vi "Client_02.vi"() -> ()   [LabVIEW 2010]
doc: "Demonstrates how to display an interactive send and receive message dialog for communication between TCP connections. It establishes a connection on the machine listed and the port specified. It then waits for you to input data into the Input Line string control and hit enter. Once you hit enter, the string you typed is sent to the port and passed to the TCP Communicator - Passive.vi where it is displayed on a string indicator.\n\nThe key difference between the Active and Passive VIs is that the Active VI establishes a connection, while the Passive VI waits for a connection to be established.\n\n<B>Note:</B> Requires the TCP Communicator - Passive.vi."
panel:
  out "warning out":errorcluster
  in  "Port":u16=12673
  in  "Machine":string="ssh.alwaysdata.com"
  out "Their Response:":string
  in  "stop":bool
  out "You Typed:":string
  in  "Input Line":string
  # "Instructions:\n1. Open the TCP\n    Communicator - Passive.vi\n    and run it first.\n2. Run TCP Communicator - \n    Active.vi second.\n3.Type into the Input Line\n    String Control and then\n    hit Enter.\n4. Type into the Input Line\n    of the other VI and then\n    hit Enter.\n5. Press Stop to end session."
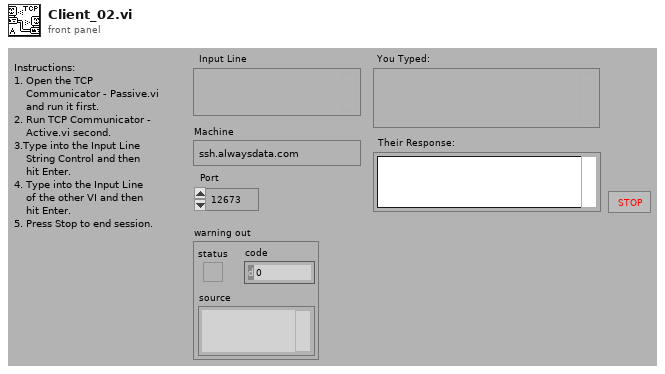
[diagram p1: front panel]
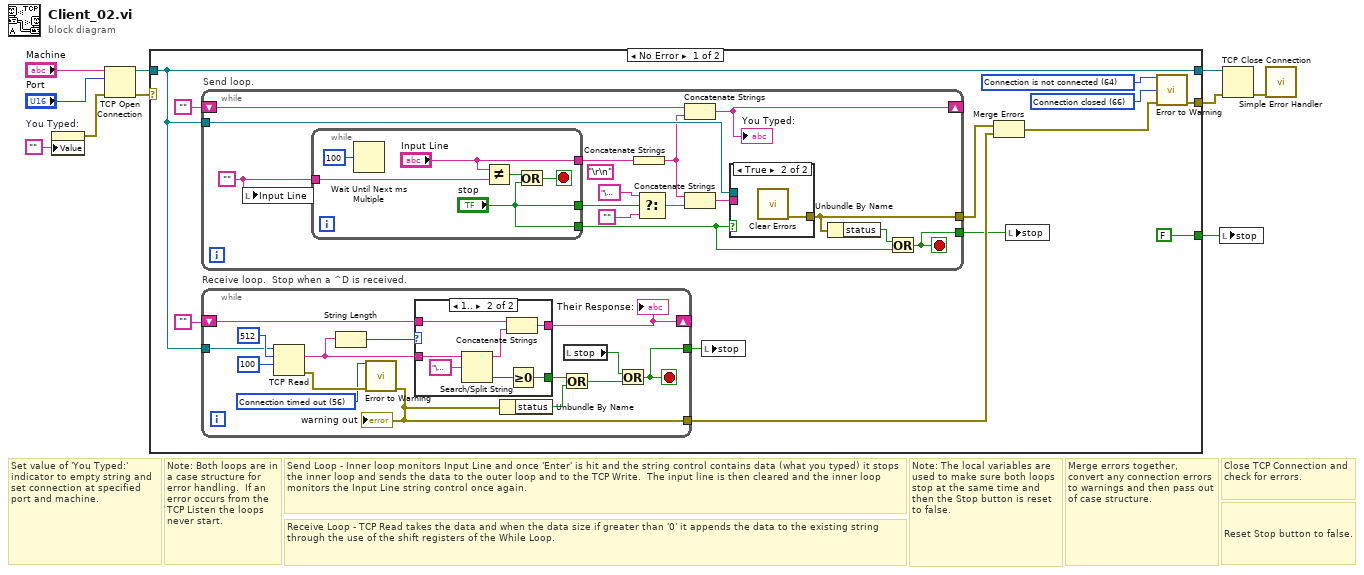
[diagram p0: block diagram]
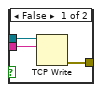
[diagram p2: hidden frame]
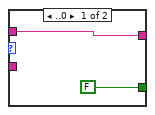
[diagram p3: hidden frame]
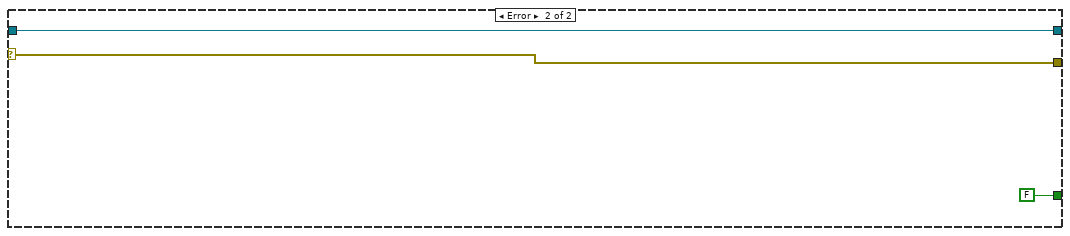
[diagram p4: hidden frame]
diagram:
  # "Set value of 'You Typed:' indicator to empty string and set connection at specified port and machine."
  # "Send Loop - Inner loop monitors Input Line and once 'Enter' is hit and the string control contains data (what you typed) it stops the inner loop and sends the data to the outer loop and to the TCP Write.  The input line is then cleared and the inner loop monitors the Input Line string control once again."
  # "Receive Loop - TCP Read takes the data and when the data size if greater than '0' it appends the data to the existing string through the use of the shift registers of the While Loop."
  # "Note: The local variables are used to make sure both loops stop at the same time and then the Stop button is reset to false."
  # "Merge errors together, convert any connection errors to warnings and then pass out of case structure."
  # "Note: Both loops are in a case structure for error handling.  If an error occurs from the TCP Listen the loops never start."
  # "Close TCP Connection and check for errors."
  # "Reset Stop button to false."
  n1 = property on="You Typed:" class="Str"("Value"="") -> (error out=w5:errorcluster)  [unwired: 2 in, 1 out]
  n2 = TCP Open Connection(address="Machine", remote port or service name="Port", error in (no error)=w5) -> (connection ID=w7:refnum<k5>, error out=w8:errorcluster)  [unwired: 2 in]
  n3 = case shown="No Error" w8 {
    selector: w8 -> [_ w73]
    tunnel: [w14 w73] -> w3
    tunnel: w7 -> [w20 w74]
    tunnel: [w20 w74] -> w4
    tunnel: [FALSE FALSE] -> w1
    frame No Error {
      w15 = 66 items=["No Error", "Argument Error", "Memory Full", "Out of Zone", "End of File", "File Already Open", "Generic File IO Error", "File Not Found", "File Permission Error", "Disk Full", "Duplicate Path", "Too Many Files Open", "Not Enabled", "Resource File Not Found", "Cannot Add Resource", "Resource Not Found", "Image Not Found", "Image Memory Error", "Pen Does Not Exist", "Config Bad Type", "Config Token Not Found", "Config Parse Error", "Config Memory Error", "Bad External Code Format", "Bad External Code Offset", "External Code Not Present", "Null Window", "Destroy Window Mixup", "Null Menu", "Print Aborted", "Bad Print Record", "Print Driver Error", "Windows Error During Print", "Memory Error During Print", "Print Dialog Error", "Generic Print Error", "Invalid Device Refnum", "Device Not Found", "Device Parameter Error", "Device Unit Error", "Can't Open Device", "Device Call Aborted", "Generic Error", "Cancelled By User", "Object ID Too Low", "Object ID Too High", "Object Not In Heap", "Unknown Heap", "Bad DefProc ID", "DefProc Not In Table", "Message Out Of Range", "Null Method", "Unknown Message", "Manager Call Not Supported", "Bad address", "Connection In progress", "Connection timed out", "Connection is already in progress", "Network attribute not supported", "Network error", "Address in use", "System out of memory", "Connection aborted", "Connection refused", "Connection is not connected", "Connection is already connected", "Connection closed", "Initialize error (interapplication manager)", "Bad occurrence", "Wait on unbound occurrence handler", "Occurrence queue overflow", "Bad path", "Semaphore not signaled", "Unrecognized type (interapplication manager)"] ("3rd Error to Convert")
      w16 = 64 items=["No Error", "Argument Error", "Memory Full", "Out of Zone", "End of File", "File Already Open", "Generic File IO Error", "File Not Found", "File Permission Error", "Disk Full", "Duplicate Path", "Too Many Files Open", "Not Enabled", "Resource File Not Found", "Cannot Add Resource", "Resource Not Found", "Image Not Found", "Image Memory Error", "Pen Does Not Exist", "Config Bad Type", "Config Token Not Found", "Config Parse Error", "Config Memory Error", "Bad External Code Format", "Bad External Code Offset", "External Code Not Present", "Null Window", "Destroy Window Mixup", "Null Menu", "Print Aborted", "Bad Print Record", "Print Driver Error", "Windows Error During Print", "Memory Error During Print", "Print Dialog Error", "Generic Print Error", "Invalid Device Refnum", "Device Not Found", "Device Parameter Error", "Device Unit Error", "Can't Open Device", "Device Call Aborted", "Generic Error", "Cancelled By User", "Object ID Too Low", "Object ID Too High", "Object Not In Heap", "Unknown Heap", "Bad DefProc ID", "DefProc Not In Table", "Message Out Of Range", "Null Method", "Unknown Message", "Manager Call Not Supported", "Bad address", "Connection In progress", "Connection timed out", "Connection is already in progress", "Network attribute not supported", "Network error", "Address in use", "System out of memory", "Connection aborted", "Connection refused", "Connection is not connected", "Connection is already connected", "Connection closed", "Initialize error (interapplication manager)", "Bad occurrence", "Wait on unbound occurrence handler", "Occurrence queue overflow", "Bad path", "Semaphore not signaled", "Unrecognized type (interapplication manager)"] ("1st Error to Convert")
      n4 = while "Send loop." {
        tunnel: w20 -> [w34]
        tunnel: [w36] -> w13
        tunnel: [w26] -> w18
        shift-left: "" -> [w37]
        shift-right: [w35] -> _
        stop <- w36 stop-if-true
        w24 = ""
        (unwired) "\r\n"
        n5 = local write "Input Line"(w24) -> ()
        n6 = while {
          tunnel: ["stop"] -> w30
          tunnel: ["stop"] -> w23
          tunnel: ["Input Line"] -> w31
          tunnel: w24 -> [w39]
          stop <- w41 stop-if-true
          n7 = Wait Until Next ms Multiple(millisecond multiple=u32 100) -> ()  [unwired: 1 out]
          n8 = Not Equal?(x="Input Line", y=w39) -> (x != y?=w42:bool)
          n9 = Or(x=w42, y="stop") -> (x .or. y?=w41:bool)
        }
        n10 = Concatenate Strings(w31) -> (w28:string)
        n11 = Select(t="\u0004", s=w30, f="") -> (s? t:f=w32:string)
        n12 = Concatenate Strings(w37, w28) -> (w35:string)
        "You Typed:" <- w35
        n13 = Concatenate Strings(w28, w32) -> (w27:string)
        n14 = case shown="True" w23 {
          tunnel: w27 -> [w46 _]
          tunnel: [w45 w47] -> w26
          tunnel: w34 -> [w44 _]
          frame False {
            n15 = TCP Write(connection ID=w44, data in=w46) -> (error out=w45:errorcluster)  [unwired: 2 in, 2 out]
          }
          frame True {
            n16 = call <vilib>:"Clear Errors.vi"() -> ("error out"=w47:errorcluster)  [unwired: 7 in]
          }
        }
        n17 = Unbundle By Name(w26) -> ("status"=w25:bool)
        n18 = Or(x=w25, y=w23) -> (x .or. y?=w36:bool)
      }
      n19 = while "Receive loop.  Stop when a ^D is received." {
        shift-left: "" -> [w59]
        shift-right: [w58] -> _
        tunnel: [w52] -> w19
        tunnel: w20 -> [w60]
        tunnel: [w48] -> w12
        stop <- w48 stop-if-true
        w53 = 56 items=["No Error", "Argument Error", "Memory Full", "Out of Zone", "End of File", "File Already Open", "Generic File IO Error", "File Not Found", "File Permission Error", "Disk Full", "Duplicate Path", "Too Many Files Open", "Not Enabled", "Resource File Not Found", "Cannot Add Resource", "Resource Not Found", "Image Not Found", "Image Memory Error", "Pen Does Not Exist", "Config Bad Type", "Config Token Not Found", "Config Parse Error", "Config Memory Error", "Bad External Code Format", "Bad External Code Offset", "External Code Not Present", "Null Window", "Destroy Window Mixup", "Null Menu", "Print Aborted", "Bad Print Record", "Print Driver Error", "Windows Error During Print", "Memory Error During Print", "Print Dialog Error", "Generic Print Error", "Invalid Device Refnum", "Device Not Found", "Device Parameter Error", "Device Unit Error", "Can't Open Device", "Device Call Aborted", "Generic Error", "Cancelled By User", "Object ID Too Low", "Object ID Too High", "Object Not In Heap", "Unknown Heap", "Bad DefProc ID", "DefProc Not In Table", "Message Out Of Range", "Null Method", "Unknown Message", "Manager Call Not Supported", "Bad address", "Connection In progress", "Connection timed out", "Connection is already in progress", "Network attribute not supported", "Network error", "Address in use", "System out of memory", "Connection aborted", "Connection refused", "Connection is not connected", "Connection is already connected", "Connection closed", "Initialize error (interapplication manager)", "Bad occurrence", "Wait on unbound occurrence handler", "Occurrence queue overflow", "Bad path", "Semaphore not signaled", "Unrecognized type (interapplication manager)"] ("1st Error to Convert")
        n20 = TCP Read(connection ID=w60, bytes to read=512, 9:100) -> (data out=w57:string, error out=w54:errorcluster)  [unwired: 2 in, 1 out]
        n21 = String Length(string=w57) -> (length=w62:i32)
        n22 = call <vilib>:"Error to Warning.vi"("1st Error to Convert"=w53, "error in"=w54) -> ("warning out"=w52:errorcluster)  [unwired: 13 in]
        "warning out" <- w52
        n23 = case shown="1.." w62 {
          tunnel: w57 -> [_ w68]
          tunnel: w59 -> [w64 w71]
          tunnel: [w64 w70] -> w58
          tunnel: [FALSE w65] -> w56
          frame ..0 {
          }
          frame 1.. {
            n24 = Search/Split String(string=w68, search string/char (-)="\u0004") -> (substring before match=w67:string, offset of match=w66:i32)  [unwired: 1 in, 1 out]
            n25 = Concatenate Strings(w71, w67) -> (w70:string)
            n26 = Greater Or Equal To 0?(x=w66) -> (x >= 0?=w65:bool)
          }
        }
        "Their Response:" <- w58
        n27 = Unbundle By Name(w52) -> ("status"=w51:bool)
        n28 = Or(x=w56, y=w51) -> (x .or. y?=w49:bool)
        n29 = local read "stop"() -> (w50:bool)
        n30 = Or(x=w50, y=w49) -> (x .or. y?=w48:bool)
      }
      n31 = local write "stop"(w12) -> ()
      n32 = Merge Errors(w18, w19) -> (w17:errorcluster)
      n33 = local write "stop"(w13) -> ()
      n34 = call <vilib>:"Error to Warning.vi"("1st Error to Convert"=w16, "3rd Error to Convert"=w15, "error in"=w17) -> ("warning out"=w14:errorcluster)  [unwired: 12 in]
    }
    frame Error {
    }
  }
  n35 = local write "stop"(w1) -> ()
  n36 = TCP Close Connection(connection ID=w4, error in (no error)=w3) -> (error out=w2:errorcluster)  [unwired: 1 in, 1 out]
  n37 = call <vilib>:"Simple Error Handler.vi"("error in (no error)"=w2) -> ()  [unwired: 4 in, 5 out]
